vi "WordDoc.vi"(8 "error in":errorcluster) -> (0 "error out":errorcluster)   [LabVIEW 2019]
uses:
  <vilib>/Utility/NIReport.llb/Report Type.ctl
  <vilib>/Utility/NIReport.llb/Append Text Table to Report (wrap).vi
  <vilib>/Utility/NIReport.llb/NI_report.lvclass
  <vilib>/addons/_office/NI_ReportGenerationToolkit.lvlib
  <vilib>/Utility/NIReport.llb/NI_ReportGenerationCore.lvlib
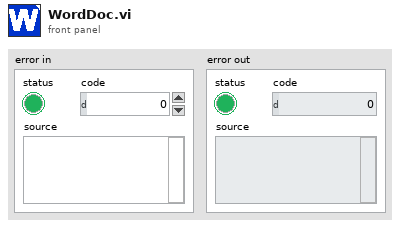
[diagram p1: front panel]
types:
  T1 = typedef "NI_ReportGenerationCore.lvlib/Report Type.ctl" = enum16{"HTML", "Word", "Excel"}
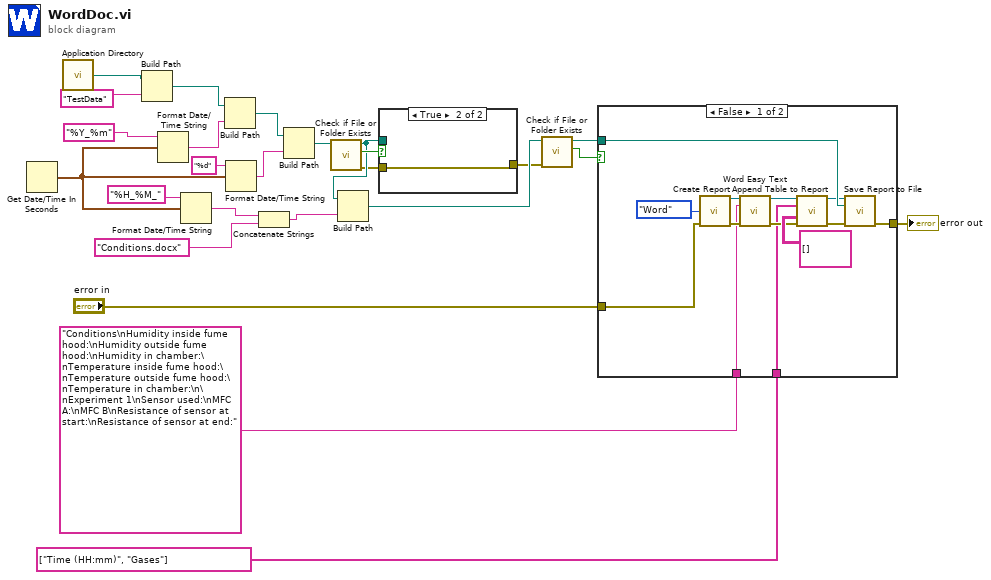
[diagram p0: block diagram]
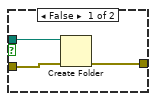
[diagram p2: hidden frame]
diagram:
  n1 = Get Date/Time In Seconds() -> (seconds since 1Jan1904=w9:timestamp)
  n2 = call <vilib>:"Application Directory.vi"() -> ("Application Directory"=w25:path)
  n3 = Build Path(base path=w25, name or relative path="TestData") -> (appended path=w21:path)
  n4 = Format Date/Time String(time format string (%c)="%Y_%m", seconds (now)=w9) -> (date/time string=w22:string)  [unwired: 1 in]
  n5 = Format Date/Time String(time format string (%c)="%H_%M_", seconds (now)=w9) -> (date/time string=w10:string)  [unwired: 1 in]
  n6 = Build Path(base path=w21, name or relative path=w22) -> (appended path=w20:path)
  n7 = Format Date/Time String(time format string (%c)="%d", seconds (now)=w9) -> (date/time string=w18:string)  [unwired: 1 in]
  n8 = Concatenate Strings(w10, "Conditions.docx" ("name or relative path")) -> (w7:string)
  n9 = Build Path(base path=w20, name or relative path=w18) -> (appended path=w6:path)
  n10 = call <vilib>:"Check if File or Folder Exists.vi"("path"=w6) -> ("error out"=w3:errorcluster, "file or folder exists?"=w5:bool, "dup path"=w4:path)  [unwired: 8 in]
  n11 = Build Path(base path=w4, name or relative path=w7) -> (appended path=w17:path)
  n12 = case shown="True" w5 {
    tunnel: w4 -> [w28 _]
    tunnel: w3 -> [w27 w29]
    tunnel: [w26 w29] -> w2
    frame False {
      n13 = Create Folder(path (use dialog)=w28, error in=w27) -> (error out=w26:errorcluster)  [unwired: 1 in, 2 out]
    }
    frame True {
    }
  }
  n14 = call <vilib>:"Check if File or Folder Exists.vi"("error in (no error)"=w2, "path"=w17) -> ("file or folder exists?"=w1:bool, "dup path"=w14:path)  [unwired: 7 in, 1 out]
  n15 = case shown="False" w1 {
    tunnel: "error in" -> [w33 w43]
    tunnel: [w38 w43] -> w15
    tunnel: w14 -> [w40 _]
    tunnel: "Conditions\nHumidity inside fume hood:\nHumidity outside fume hood:\nHumidity in chamber:\nTemperature inside fume hood:\nTemperature outside fume hood:\nTemperature in chamber:\n\nExperiment 1\nSensor used:\nMFC A:\nMFC B\nResistance of sensor at start:\nResistance of sensor at end:" ("text") -> [w37 _]
    tunnel: string[] ["Time (HH:mm)", "Gases"] ("column headers") -> [w31 _]
    frame False {
      n16 = call <vilib>:"Create Report.vi"("report type"=Report_Type."Word", "error in (no error)"=w33) -> ("report out"=w42:refnum<class "NI_report.lvclass">, "error out"=w39:errorcluster)  [unwired: 12 in]
      n17 = call <vilib>:"Word Easy Text.vi"("report in"=w42, "text"=w37, "error in (no error)"=w39) -> ("report out"=w36:refnum<class "NI_report.lvclass">, "error out"=w32:errorcluster)  [unwired: 10 in, 1 out]
      n18 = call-poly <vilib>:"Append Table to Report.vi"("report in"=w36, "column headers"=w31, "text data"=string[][] [], "error in (no error)"=w32) -> ("report out"=w35:refnum<class "NI_report.lvclass">, "error out"=w30:errorcluster)  [unwired: 8 in, 2 out]
      n19 = call-dynamic "Save Report to File.vi"("report in"=w35, "report file path"=w40, "error in (no error)"=w30) -> ("error out"=w38:errorcluster)  [unwired: 11 in, 1 out]
    }
    frame True {
    }
  }
  "error out" <- w15
